vi "GetRawWaveform.vi"(8 "error in (no error)":errorcluster, 10 "Byte Size per point (1 byte)":i32=1 min=1 max=2, 11 "VISA Resource Name":refnum<visa-resource-name>) -> (0 "error out":errorcluster, 1 "Waveform Array":i16[](array[numeric]), 3 "VISA Resource Name Out":refnum<visa-resource-name>)   [LabVIEW 2010, in "Tektronix TDS 3000 Series.lvlib"]
doc: "This VI acquires the raw unscaled waveform that the oscilliscope sends back."
uses:
  <instrlib>/Tektronix TDS 3000 Series/Tektronix TDS 3000 Series.lvlib
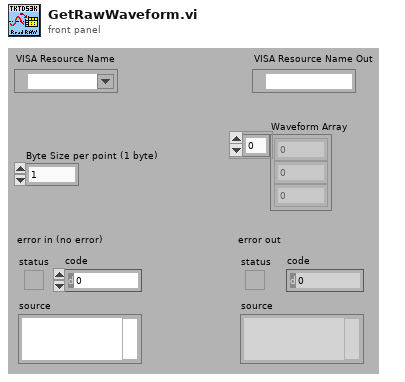
[diagram p1: front panel]
types:
  T1 = cluster{"status":bool, "error code (0)":i32, "source":string}
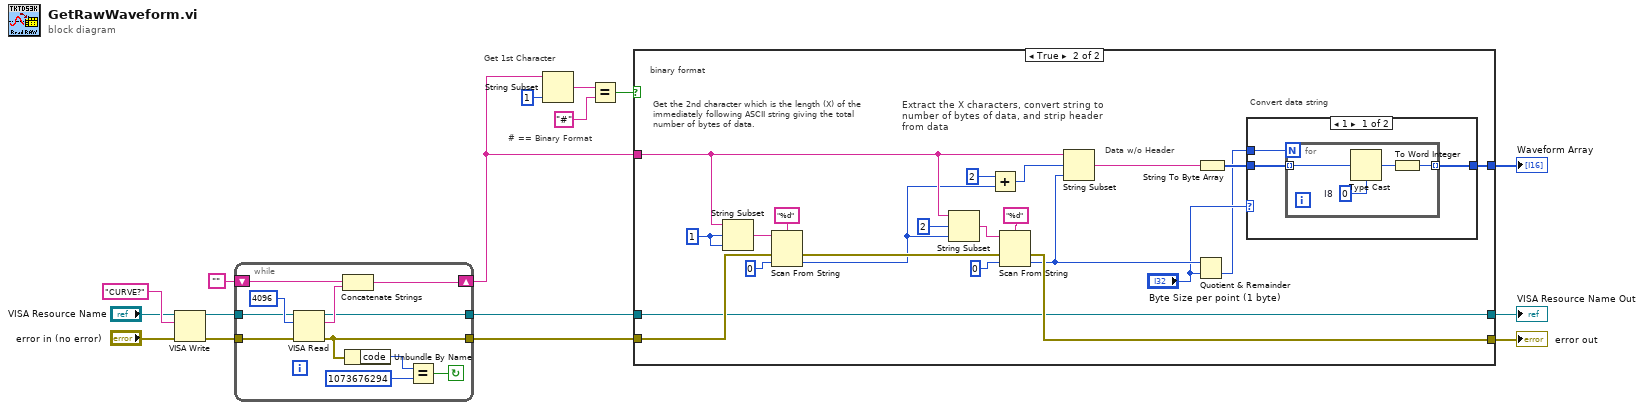
[diagram p0: block diagram]
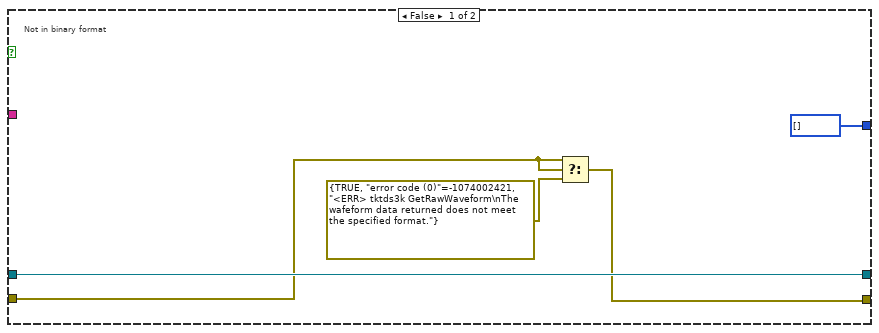
[diagram p2: hidden frame]
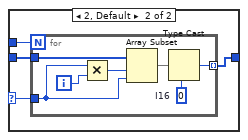
[diagram p3: hidden frame]
diagram:
  # "# == Binary Format"
  # "Get 1st Character"
  n1 = VISA Write(VISA resource name="VISA Resource Name", write buffer="CURVE?" ("Command"), error in (no error)="error in (no error)") -> (VISA resource name out=w5:refnum<visa-resource-name>, error out=w4:errorcluster)  [unwired: 1 out]
  n2 = while {
    tunnel: [w18] -> w1
    tunnel: w4 -> [w20]
    shift-left: "" -> [w23]
    shift-right: [w21] -> w3
    tunnel: w5 -> [w24]
    tunnel: [w17] -> w2
    stop <- w19 continue-if-true
    n3 = VISA Read(VISA resource name=w24, byte count=u32 4096 ("byte count (0)"), error in (no error)=w20) -> (VISA resource name out=w17:refnum<visa-resource-name>, read buffer=w22:string, error out=w18:errorcluster)  [unwired: 1 out]
    n4 = Concatenate Strings(w23, w22) -> (w21:string)
    n5 = Unbundle By Name(w18) -> ("code"=w26:i32)
    n6 = Equal?(x=w26, y=1073676294 ("x")) -> (x = y?=w19:bool)
  }
  n7 = String Subset(string=w3, length (rest)=1 ("length (rest)")) -> (substring=w13:string)  [unwired: 1 in]
  n8 = Equal?(x=w13, y="#" ("First Char")) -> (x = y?=w11:bool)
  n9 = case shown="True" w11 {
    tunnel: [w30 w42] -> w8
    tunnel: [i16[] [] ("unsigned byte array") w43] -> w15
    tunnel: w3 -> [_ w49]
    tunnel: w1 -> [w29 w51]
    tunnel: [w32 w41] -> w7
    tunnel: w2 -> [w32 w41]
    frame False {
      # "Not in binary format"
      n10 = Select(t=w29, s=w29, f=cluster{bool, "error code (0)":i32, string} {TRUE, "error code (0)"=-1074002421, "<ERR> tktds3k GetRawWaveform\nThe wafeform data returned does not meet the specified format."} ("output cluster")) -> (s? t:f=w30:T1)
    }
    frame True {
      w50 = 1 ("offset (0)")
      # "binary format"
      # "Get the 2nd character which is the length (X) of the immediately following ASCII string giving the total number of bytes of data."
      # "Convert data string"
      # "Extract the X characters, convert string to number of bytes of data, and strip header from data"
      # "Data w/o Header"
      n11 = String Subset(string=w49, offset (0)=w50, length (rest)=w50) -> (substring=w33:string)
      n12 = Scan From String(format string="%d", input string=w33, error in=w51, default 1=0 ("Default Value 1")) -> (error out=w52:errorcluster, output 1=w47:i32)  [unwired: 1 in, 2 out]
      n13 = String Subset(string=w49, offset (0)=2, length (rest)=w47) -> (substring=w38:string)
      n14 = Add(x=2, y=w47) -> (x+y=w46:i32)
      n15 = Scan From String(format string="%d", input string=w38, error in=w52, default 1=0 ("Default Value 1")) -> (error out=w42:errorcluster, output 1=w39:i32)  [unwired: 1 in, 2 out]
      n16 = String Subset(string=w49, offset (0)=w46, length (rest)=w39) -> (substring=w45:string)
      n17 = Quotient & Remainder(x=w39, y="Byte Size per point (1 byte)") -> (floor(x/y)=w34:i32)  [unwired: 1 out]
      n18 = String To Byte Array(string=w45) -> (unsigned byte array=w44:u8[])
      n19 = case shown="1" "Byte Size per point (1 byte)" {
        selector: "Byte Size per point (1 byte)" -> [_ w63]
        tunnel: w44 -> [w57 w65]
        tunnel: w34 -> [w55 w64]
        tunnel: [w56 w62] -> w43
        frame 1 {
          n20 = for {
            N: w55 -> [_]
            tunnel: w57 -> [w61] mode=indexing
            tunnel: [w59] -> w56 mode=indexing
            w58 = i8 0  # I8
            n21 = Type Cast(type=w58, x=w61) -> (*(type *) &x=w60:i8)
            n22 = To Word Integer(number=w60) -> (16bit integer=w59:i16)
          }
        }
        frame 2, Default {
          n23 = for {
            N: w64 -> [_]
            tunnel: w63 -> [w69]
            tunnel: [w67] -> w62 mode=indexing
            tunnel: w65 -> [w72]
            i -> [w70]
            w66 = i16 0  # I16
            n24 = Multiply(x=w69, y=w70) -> (x*y=w71:i32)
            n25 = Array Subset(array=w72, index=w71, length=w69) -> (w68:u8[])
            n26 = Type Cast(type=w66, x=w68) -> (*(type *) &x=w67:i16)
          }
        }
      }
    }
  }
  "Waveform Array" <- w15
  "error out" <- w8
  "VISA Resource Name Out" <- w7
